vi "Test Draw To Picture Greyscale.vi"(8 "error in (no error)":errorcluster, 11 "Test Case In":refnum<class "01_Image.lvclass">) -> (0 "error out":errorcluster, 3 "Test Case Out":refnum<class "01_Image.lvclass">)   [LabVIEW 2020, in "test.lvlib" / "01_Image.lvclass"]
uses:
  01_Image.lvclass
  C:/Program Files (x86)/National Instruments/LabVIEW 2026/vi.lib/Astemes/LUnit/Test Case.lvclass
  image/Image Draw Offset.ctl
  common/Image Size (Integer).ctl
  <vilib>/Astemes/LUnit/Test Case.lvclass/Test Case.ctl
  4993e8ee-a06a-463a-9684-69129f64d5ce.vi
  image/New Image.vi
  image/New Image (Greyscale Preallocated).vi
  image/Copy Array to Image.vi
  image/Copy Array to Image (Greyscale).vi
  image/Draw Image to Picture (Greyscale).vi/9ae995ca-ccda-485c-89ac-02736fde3e8e.vi
  <vilib>/Astemes/LUnit/Core/LUnit Test Case/Private/Append Pass Result.vi
  <vilib>/Astemes/LUnit/Core/LUnit Test Case/Private/Append Fail Result.vi
  4993e8ee-a06a-463a-9684-69129f64d5ce.vi/9c5d11cd-9439-4240-a1ee-d9baace9c924.vi
  image/New Image (Greyscale Preallocated).vi/6598b9e0-8a08-46f5-91fd-ca1b87217137.vi
  <vilib>/Astemes/LUnit/Core/LUnit Test Case/Private/Run In UI.vi
  <vilib>/Utility/error.llb/Clear Errors.vi
  <vilib>/Utility/error.llb/Error Cluster From Error Code.vi
  image/image.lvlib
  common/common.lvlib
panel:
  out "Actual":picture
  out "Expected":picture
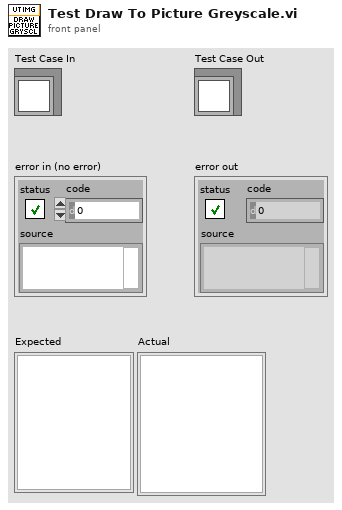
[diagram p1: front panel]
types:
  T1 = typedef "common.lvlib/Image Size (Integer).ctl" = cluster{"Width":u16, "Height":u16}
  T2 = typedef "image.lvlib/Image Draw Offset.ctl" = cluster{"Left":i16, "Top":i16}
  T3 = typedef "image.lvlib/Greyscale Image.ctl" = refnum<data-value>
  T4 = typedef "imagedata.ctl" = cluster{"image type":i32, "image depth":i32, "image":u8[], "mask":u8[], "colors":u32[], "Rectangle":cluster{"left":i16, "top":i16, "right":i16, "bottom":i16}}
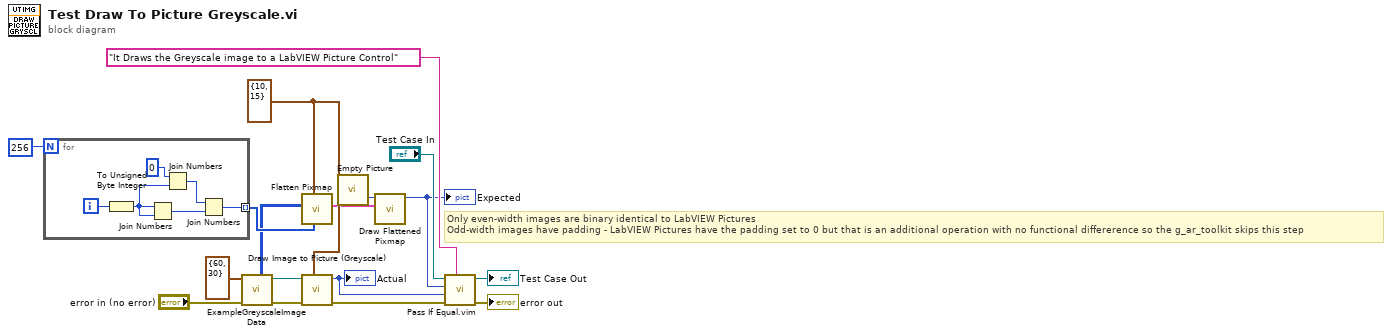
[diagram p0: block diagram]
diagram:
  w12 = T2 {"Left"=10, "Top"=15} ("Top-Left (0,0)")
  # "Only even-width images are binary identical to LabVIEW Pictures\nOdd-width images have padding - LabVIEW Pictures have the padding set to 0 but that is an additional operation with no functional differerence so the g_ar_toolkit skips this step"
  n1 = for {
    N: 256 -> [_]
    tunnel: [w22] -> w8 mode=indexing
    i -> [w23]
    n2 = To Unsigned Byte Integer(number=w23) -> (unsigned 8bit integer=w19:u8)
    n3 = Join Numbers(hi=w19, lo=w19) -> ((hi.lo)=w21:u16)
    n4 = Join Numbers(hi=u8 0, lo=w19) -> ((hi.lo)=w20:u16)
    n5 = Join Numbers(hi=w20, lo=w21) -> ((hi.lo)=w22:u32)
  }
  n6 = call "ExampleGreyscaleImageData.vi"("error in (no error)"="error in (no error)", "Image Size"=T1 {"Width"=60, "Height"=30}) -> ("error out"=w4:errorcluster, "Greyscale Destination Image"=w3:T3, "Greyscale Data"=w2:u8[][])  [unwired: 6 in, 1 out]
  n7 = call <vilib>:"Flatten Pixmap.vi"("colors"=w8, "top left"=w12, "8-bit pixmap"=w2) -> ("image data"=w11:T4)  [unwired: 8 in]
  n8 = call "Draw Image to Picture (Greyscale).vi"("Image Draw Offset (Default 0,0)"=w12, "error in (no error)"=w4, "Greyscale Image Source in"=w3) -> ("error out"=w13:errorcluster, "Picture"=w6:picture)  [unwired: 7 in]
  "Actual" <- w6
  n9 = call "Empty Picture"() -> ("empty picture"=w10:picture)
  n10 = call <vilib>:"Draw Flattened Pixmap.vi"("image data"=w11, "picture"=w10) -> ("new picture"=w7:picture)  [unwired: 7 in]
  "Expected" <- w7
  n11 = call "Pass If Equal.vim"("Description"="It Draws the Greyscale image to a LabVIEW Picture Control", "error in (no error)"=w13, "Actual"=w6, "Expected"=w7, "LUnit Test Case In"="Test Case In") -> ("error out"=→"error out":errorcluster, "LUnit Test Case Out"=→"Test Case Out":refnum<class "01_Image.lvclass">)  [unwired: 5 in]
